vi "CODCr操作日志.vi"(11 "data in":T1) -> ()   [LabVIEW 2016, in "CODCr库.lvlib"]
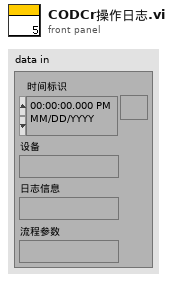
[diagram p1: front panel]
types:
  T1 = cluster{"时间标识":timestamp, "设备":string, "日志信息":string, "流程参数":string}
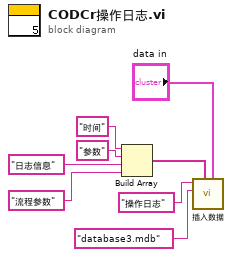
[diagram p0: block diagram]
diagram:
  n1 = Build Array("时间", "参数" ("元素"), "日志信息", "流程参数") -> (w3:string[])
  n2 = call "插入数据.vi"("data"="data in", "columns"=w3, "database"="database3.mdb", "table"="操作日志") -> ()  [unwired: 7 in, 1 out]
